vi "endPlay.vi"(8 "error in (no error)":errorcluster, 11 "Football in":refnum<class "Football.lvclass">) -> (0 "error out":errorcluster, 3 "Football out":refnum<class "Football.lvclass">)   [LabVIEW 2018, in "Football.lvclass"]
uses:
  Football.lvclass
  ConsoleOut/Print Options.ctl
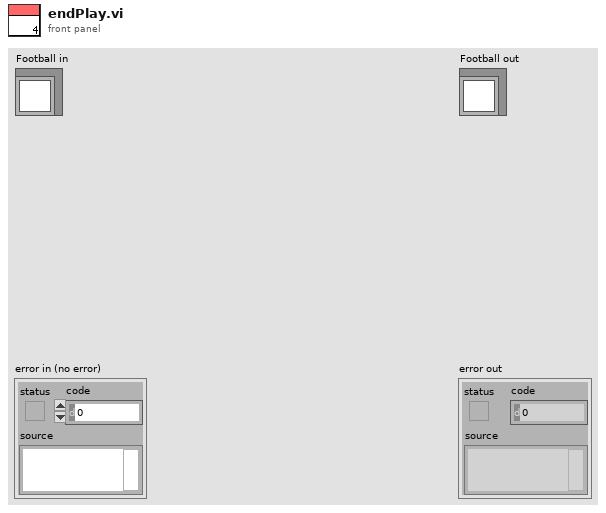
[diagram p1: front panel]
types:
  T1 = typedef "Print Options.ctl" = enum16{"Create", "Get Reference", "Print", "Print Header", "Close"}
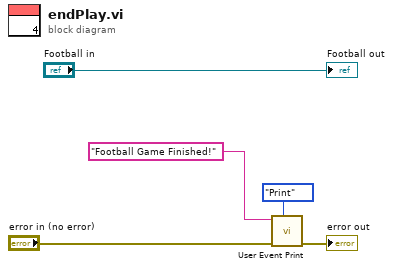
[diagram p0: block diagram]
diagram:
  n1 = call "User Event Print.vi"("Options"=Print_Options."Print", "error in (no error)"="error in (no error)", "String to Print"="Football Game Finished!" ("message")) -> ("error out"=→"error out":errorcluster)  [unwired: 7 in, 1 out]
  "Football out" <- "Football in"
